vi "GEOM_RCSimAllCols.vi"(9 "ROIS":T1(array[cluster]), 10 "amplifiers":T2[](array[typedef]) {"fliped" items=["none", "horizontal", "vertical"]; "type" items=["LL", "LR", "UL", "UR"]}) -> (1 "Corrected ROIs":T1(array[cluster]))   [LabVIEW 2016]
uses:
  GEOM_Amplifier.ctl
  GEOM_AmpType.ctl
  GEOM_ROI.ctl
  GEOM_Coords.ctl
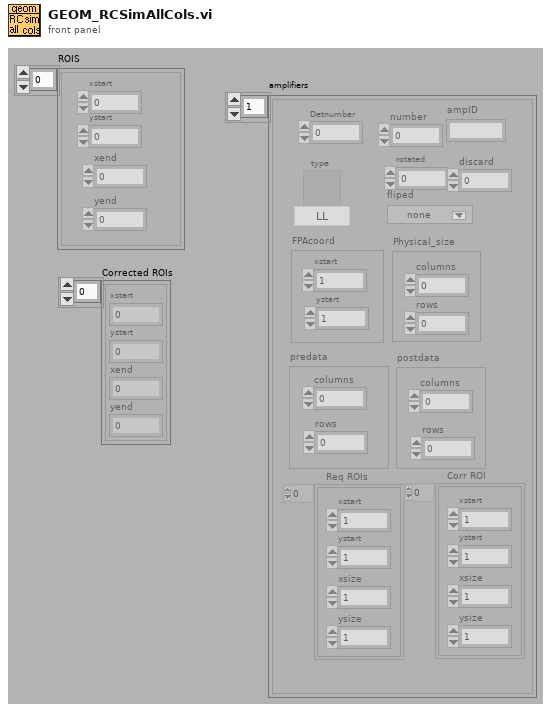
[diagram p1: front panel]
types:
  T1 = cluster{"xstart":i32, "ystart":i32, "xend":i32, "yend":i32}[]
  T2 = typedef "GEOM_Amplifier.ctl" = cluster{"number":i32, "type":T3, "rotated":i16, "fliped":u16, "FPAcoord":cluster{"xstart":i32, "ystart":i32}, "Physical_size":cluster{"columns":i32, "rows":i32}, "predata":cluster{"columns":i32, "rows":i32}, "postdata":cluster{"columns":i32, "rows":i32}, "Req ROIs":T4, "Corr ROI":T4, "Detnumber":i32, "ampID":string, "discard":i32}
  T3 = typedef "GEOM_AmpType.ctl" = u16
  T4 = typedef "GEOM_ROI.ctl" = T5[]
  T5 = typedef "GEOM_Coords.ctl" = cluster{"xstart":u32, "ystart":u32, "xsize":u32, "ysize":u32}
  T6 = cluster{"xstart":i32, "ystart":i32, "xend":i32, "yend":i32}
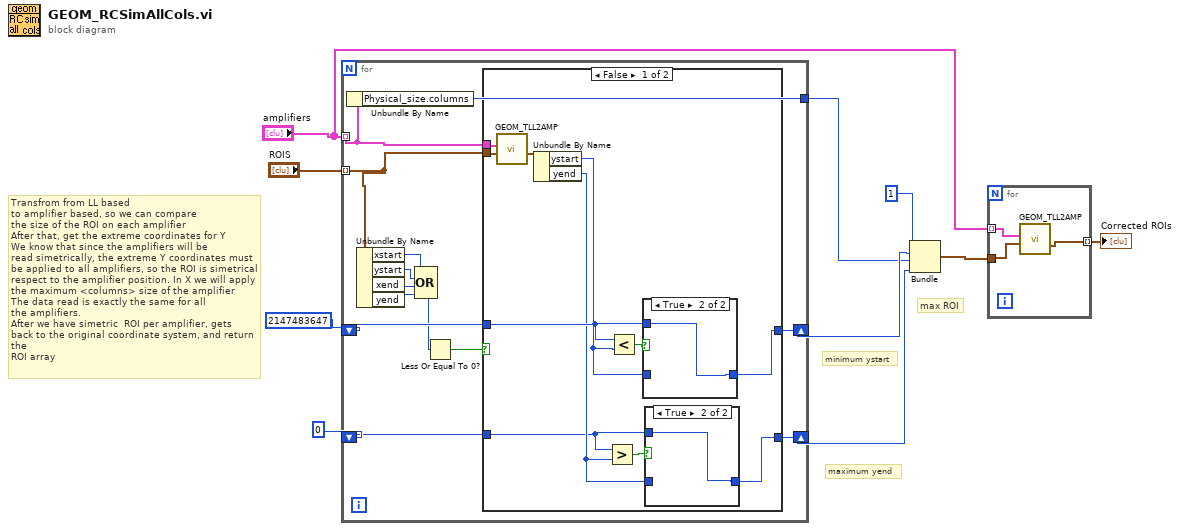
[diagram p0: block diagram]
diagram:
  # "Transfrom from LL based\nto amplifier based, so we can compare\nthe size of the ROI on each amplifier\nAfter that, get the extreme coordinates for Y\nWe know that since the amplifiers will be \nread simetrically, the extreme Y coordinates must\nbe applied to all amplifiers, so the ROI is simetrical\nrespect to the amplifier position. In X we will apply\nthe maximum <columns> size of the amplifier\nThe data read is exactly the same for all\nthe amplifiers. \nAfter we have simetric  ROI per amplifier, gets\nback to the original coordinate system, and return the\nROI array"
  # "max ROI"
  # "maximum yend"
  # "minimum ystart"
  n1 = for {
    tunnel: "ROIS" -> [w19] mode=indexing
    tunnel: "amplifiers" -> [w12] mode=indexing
    shift-right: [w23] -> w8
    shift-left: 2147483647 -> [w22]
    shift-right: [w21] -> w7
    shift-left: 0 -> [w20]
    tunnel: [w11] -> w1
    n2 = Unbundle By Name(w12) -> ("Physical_size.columns"=w11:i32)
    n3 = Unbundle By Name(w19) -> ("xstart"=w18:i32, "ystart"=w17:i32, "xend"=w16:i32, "yend"=w15:i32)
    n4 = Compound Arithmetic op=OR(w18, w17, w16, w15) -> (w14:i32)
    n5 = Less Or Equal To 0?(x=w14) -> (x <= 0?=w13:bool)
    n6 = case shown="False" w13 {
      tunnel: w12 -> [w34 _]
      tunnel: w19 -> [w33 _]
      tunnel: [w28 w40] -> w23
      tunnel: w22 -> [w27 w40]
      tunnel: [w25 w39] -> w21
      tunnel: w20 -> [w24 w39]
      frame False {
        n7 = call "GEOM_TLL2AMP.vi"("DETROIcoords"=w33, "Amplifier"=w34) -> ("AMPROICoords"=w32:T6)  [unwired: 9 out]
        n8 = Unbundle By Name(w32) -> ("ystart"=w29:i32, "yend"=w26:i32)
        n9 = Greater?(x=w24, y=w26) -> (0:w31:bool)
        n10 = Less?(x=w27, y=w29) -> (x < y?=w30:bool)
        n11 = case shown="True" w30 {
          tunnel: w29 -> [w37 _]
          tunnel: [w37 w38] -> w28
          tunnel: w27 -> [_ w38]
          frame False {
          }
          frame True {
          }
        }
        n12 = case shown="True" w31 {
          tunnel: w26 -> [w35 _]
          tunnel: [w35 w36] -> w25
          tunnel: w24 -> [_ w36]
          frame False {
          }
          frame True {
          }
        }
      }
      frame True {
      }
    }
  }
  n13 = Bundle(1, w8, "columns"=w1, w7) -> (w6:cluster{i32, i32, "columns":i32, i32})  [unwired: 1 out]
  n14 = for {
    tunnel: w6 -> [w41]
    tunnel: "amplifiers" -> [w43] mode=indexing
    tunnel: [w42] -> w4 mode=indexing
    n15 = call "GEOM_TLL2AMP.vi"("DETROIcoords"=w41, "Amplifier"=w43) -> ("AMPROICoords"=w42:T6)  [unwired: 9 out]
  }
  "Corrected ROIs" <- w4
